vi "half adder and full adder.vi"() -> ()   [LabVIEW 2013]
panel:
  out "Boolean 5":bool
  out "Boolean 4":bool
  in  "Boolean 3":bool
  in  "Boolean 2":bool
  in  "Boolean":bool
  out "carrry":bool
  out "sum":bool
  in  "a":bool
  in  "b":bool
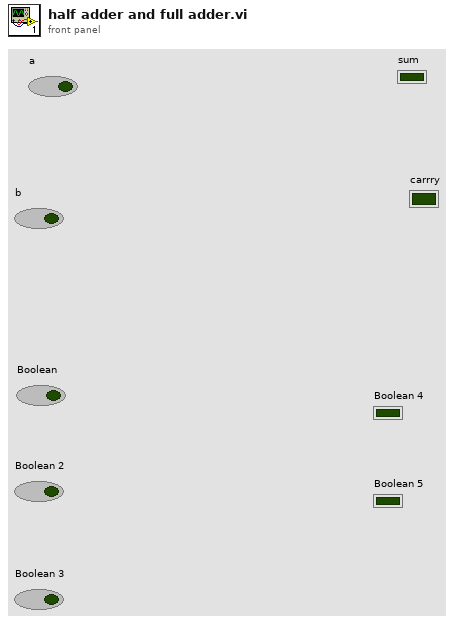
[diagram p1: front panel]
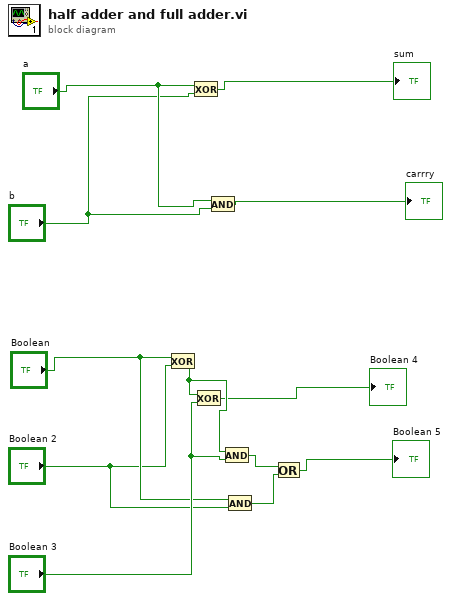
[diagram p0: block diagram]
diagram:
  n1 = Exclusive Or(1:"Boolean 2", 2:"Boolean") -> (0:w8:bool)
  n2 = Exclusive Or(1:"b", 2:"a") -> (0:→"sum":bool)
  n3 = Exclusive Or(1:"Boolean 3", 2:w8) -> (0:→"Boolean 4":bool)
  n4 = And(x="a", y="b") -> (x .and. y?=→"carrry":bool)
  n5 = And(x=w8, y="Boolean 3") -> (x .and. y?=w4:bool)
  n6 = And(x="Boolean", y="Boolean 2") -> (x .and. y?=w3:bool)
  n7 = Or(x=w4, y=w3) -> (x .or. y?=→"Boolean 5":bool)
